vi "Ching_5th_Exercise0_11-29-16.vi"   [LabVIEW 2014, in "Capucao_Ching_5th_LEGORobotics_11-29-16.lvrbt"]
uses:
  Capucao_Ching_5th_LEGORobotics_11-29-16.lvrbt
  <vilib>/NXT/Dual Mode Library/Display/drawText.vi
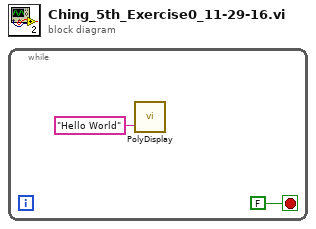
[diagram p0: block diagram]
diagram:
  n1 = while {
    stop <- FALSE stop-if-true
    n2 = call-poly <vilib>:"PolyDisplay.vi"("Text"="Hello World") -> ()  [unwired: 3 in, 1 out]
  }
